vi "Post-Build Action.vi"(5 "Files Generated by Build":path[](array[path]), 6 "Top Level/Always Included VIs":path[](array[path]), 7 "Destination Path":path, 8 "error in (no error)":errorcluster, 9 "Target Name":string, 10 "Build Specification Name":string, 11 "Project Path":path) -> (0 "error out":errorcluster)   [LabVIEW 2020]
uses:
  7012fb88-9d9e-41a1-98f5-5b23f9ff89cc.vi
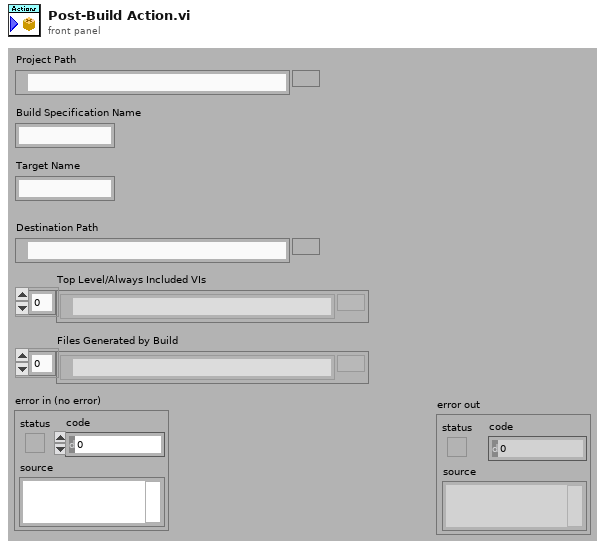
[diagram p1: front panel]
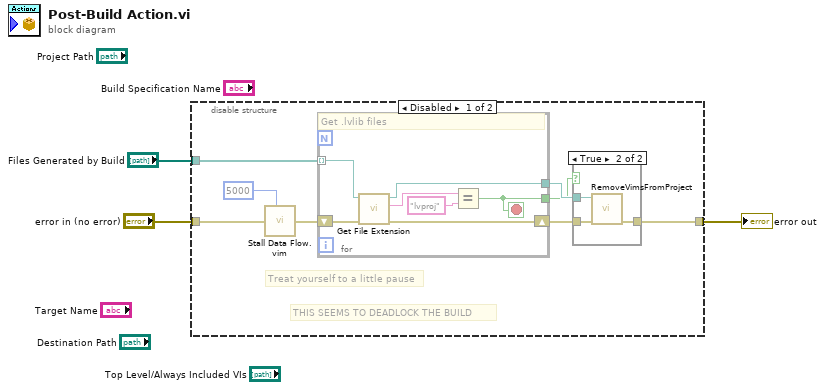
[diagram p0: block diagram]
diagram:
  n1 = disable-structure shown="Disabled" {
    disable-tunnel: "error in (no error)" -> [w11 w23]
    disable-tunnel: [w10 w23] -> w2
    disable-tunnel: "Files Generated by Build" -> [w9 _]
    frame Disabled {
      # "THIS SEEMS TO DEADLOCK THE BUILD"
      # "Treat yourself to a little pause"
      n2 = call "Stall Data Flow.vim"("value in"=w11, "milliseconds to wait"=u32 5000) -> ("value out"=w7:errorcluster)  [unwired: 1 out]
      n3 = for {
        tunnel: w9 -> [w18] mode=indexing
        shift-right: [w16] -> w5
        shift-left: w7 -> [w17]
        tunnel: [w14] -> w6
        tunnel: [w12] -> w4
        stop <- w12 stop-if-true
        # "Get .lvlib files"
        n4 = call <vilib>:"Get File Extension.vi"("error in (no error)"=w17, "file"=w18) -> ("error out"=w16:errorcluster, "lowercase file extension"=w15:string, "dup file"=w14:path)  [unwired: 5 in, 2 out]
        n5 = Equal?(x=w15, y="lvproj") -> (x = y?=w12:bool)
      }
      n6 = case shown="True" w4 {
        tunnel: w6 -> [_ w20]
        tunnel: w5 -> [w19 w22]
        tunnel: [w19 w21] -> w10
        frame False {
        }
        frame True {
          n7 = call "RemoveVimsFromProject.vi"("error in (no error)"=w22, "Project Path"=w20) -> ("error out"=w21:errorcluster)  [unwired: 9 in]
        }
      }
    }
    frame Enabled {
    }
  }
  "error out" <- w2
